vi "Create All Real-Time Message Queues.vi"(8 "error in (no error)":errorcluster) -> (0 "error out":errorcluster, 3 "Message Queues out":T1)   [LabVIEW 2017, in "Message Queue.lvlib"]
doc: "This VI creates and initializes all the message queues for your application. If your application requires more than one message queue, right-click the \"Message Queues\" constant above and select Open Type Def. Add the new Message Queue(s) to the type definition, then initialize them in this VI."
uses:
  Message Queue.lvlib
  All Real-Time Message Queues.ctl
  Message Cluster.ctl
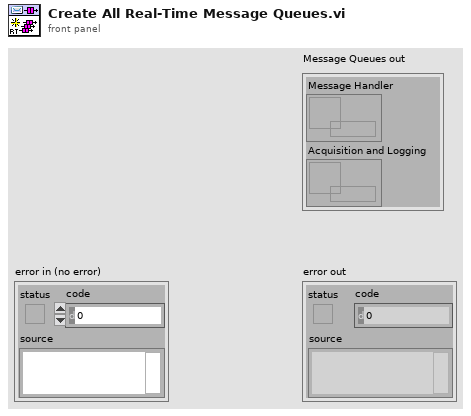
[diagram p1: front panel]
types:
  T1 = typedef "Message Queue.lvlib/All Real-Time Message Queues.ctl" = cluster{"Message Handler":refnum<queue>, "Acquisition and Logging":refnum<queue>}
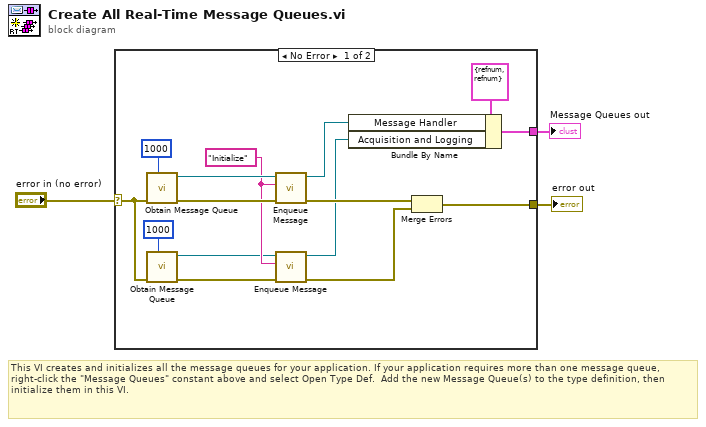
[diagram p0: block diagram]
diagram:
  # "This VI creates and initializes all the message queues for your application. If your application requires more than one message queue, right-click the \"Message Queues\" constant above and select Open Type Def.  Add the new Message Queue(s) to the type definition, then initialize them in this VI."
  n1 = case shown="No Error" "error in (no error)" {
    selector: "error in (no error)" -> [w10 w19]
    tunnel: [w12 w19] -> w3
    tunnel: [w16 _] -> w2
    frame No Error {
      w8 = "Initialize" ("Message")
      n2 = call "Obtain Message Queue.vi"("max queue size (-1, unlimited)"=1000, "error in (no error)"=w10) -> ("error out"=w15:errorcluster, "Message Queue"=w14:refnum<queue>)  [unwired: 8 in]
      n3 = call "Obtain Message Queue.vi"("max queue size (-1, unlimited)"=1000, "error in (no error)"=w10) -> ("error out"=w11:errorcluster, "Message Queue"=w7:refnum<queue>)  [unwired: 8 in]
      n4 = call "Enqueue Message.vi"("error in (no error)"=w15, "Message"=w8, "Message Queue"=w14) -> ("error out"=w18:errorcluster, "dup Message Queue"=w13:refnum<queue>)  [unwired: 7 in]
      n5 = call "Enqueue Message.vi"("error in (no error)"=w11, "Message"=w8, "Message Queue"=w7) -> ("error out"=w9:errorcluster, "dup Message Queue"=w6:refnum<queue>)  [unwired: 7 in]
      n6 = Bundle By Name(cluster=T1 {"Message Handler"=refnum, "Acquisition and Logging"=refnum} ("Message Queues"), "Message Handler"=w13, "Acquisition and Logging"=w6) -> (w16:T1)
      n7 = Merge Errors(w18, w9) -> (w12:errorcluster)
    }
    frame Error {
    }
  }
  "Message Queues out" <- w2
  "error out" <- w3
